vi "Get State.vi"(8 "error in (no error)":errorcluster, 11 "Sequencer in":refnum<class "Sequencer.lvclass">) -> (0 "error out":errorcluster, 3 "Sequencer State":T1)   [LabVIEW 2024, in "Ramses Sequencer.lvlib" / "Sequencer.lvclass"]
uses:
  Sequencer.lvclass
  C:/Program Files (x86)/Enterative/Ramses Framework/Ramses Framework.lvlibp/Service/Service.lvclass
  typedef/Sequencer State -- enum.ctl
  Program Files (x86)/Enterative/Ramses Framework/Ramses Framework.lvlibp/Service/Service.lvclass
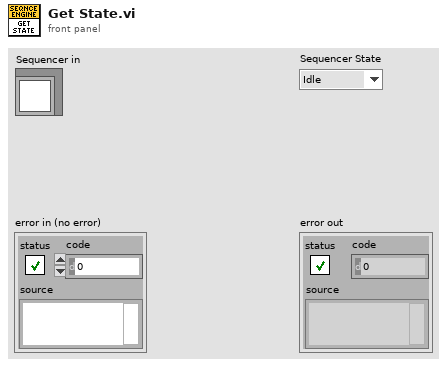
[diagram p1: front panel]
types:
  T1 = typedef "Ramses Sequencer.lvlib/Sequencer.lvclass/Sequencer State -- enum.ctl" = enum16{"Idle", "Running", "Paused", "Complete"}
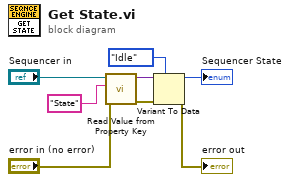
[diagram p0: block diagram]
diagram:
  n1 = call "Read Value from Property Key.vi"("error in (no error)"="error in (no error)", "Key"="State", "Service in"="Sequencer in") -> ("error out"=w3:errorcluster, "Value"=w6:variant)  [unwired: 7 in]
  n2 = Variant To Data(error in=w3, type=Sequencer_State_--_enum."Idle" ("Sequencer State"), Variant=w6) -> (data=→"Sequencer State":T1, error out=→"error out":errorcluster)
